vi "RIOTargetUI.vi"() -> ()   [LabVIEW 2014, in "RIO Target.lvclass"]
doc: "UI that will be called when the node is selected."
uses:
  RIO Target/RIO Target.lvclass
  <vilib>/NI/Configuration Framework/Node/NodeRef.ctl
  <vilib>/NI/Configuration Framework/Node/NISE_CEF_Node.lvclass
  <vilib>/NI/AMC/Message Queue.ctl
  <vilib>/NI/AMC/Message.ctl
  <vilib>/NI/Tools/Keyed Array/KeyedArray.ctl
  <vilib>/NI/Configuration Framework/Node/UserEventRef.ctl
  <vilib>/NI/Configuration Framework/Controls/EventCluster.ctl
  RIO Target/RIO Target.lvclass/RIO Target.ctl
  <vilib>/NI/Configuration Framework/serializable configuration/set metadata property.vi
  RIO Target Configuration/RIO Target Configuration.lvclass
  <vilib>/NI/Tools/Keyed Array/Tools_KeyedArray.lvlib
  <vilib>/NI/AMC/AMC.lvlib
  <vilib>/NI/Configuration Framework/NISE_CEF_TreeControl.lvlib
panel:
  out "error out":errorcluster
  in  "VI to Place Engines and IO Nodes":path
  in  "Destination Path":path
  in  "Target Project Path":path
  out "Channels per Device":string[][](table)
  in  "Generate":bool
  in  "user event":T1
  in  "main queue":T2
  in  "node ref":T3
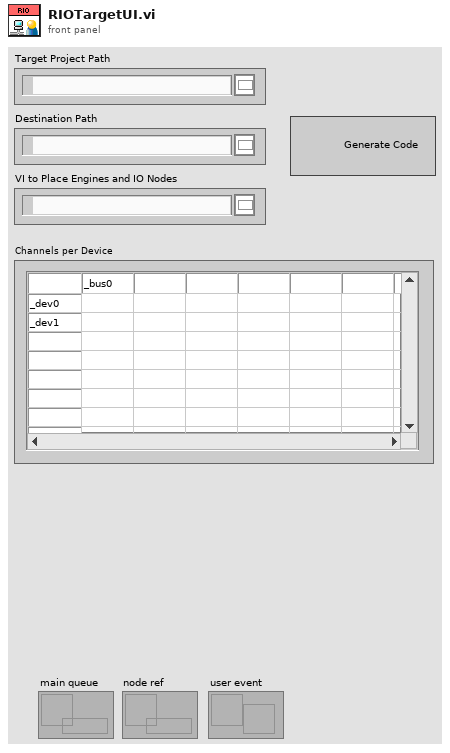
[diagram p1: front panel]
types:
  T1 = typedef "NISE_CEF_Node.lvclass/UserEventRef.ctl" = refnum<user-event>
  T2 = typedef "AMC.lvlib/Message Queue.ctl" = refnum<queue>
  T3 = typedef "NISE_CEF_Node.lvclass/NodeRef.ctl" = refnum<data-value>
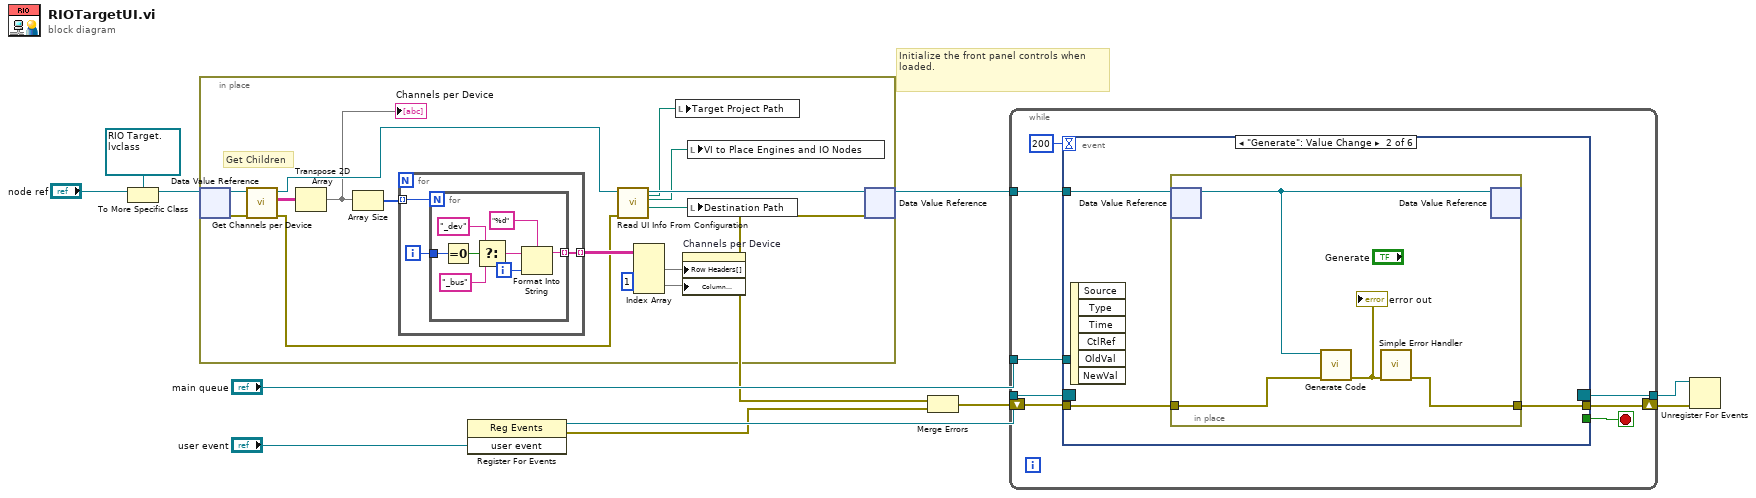
[diagram p0: block diagram]
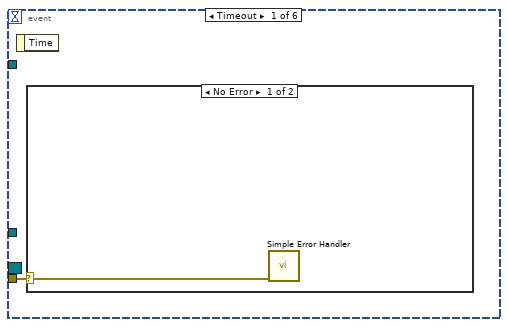
[diagram p2: hidden frame]
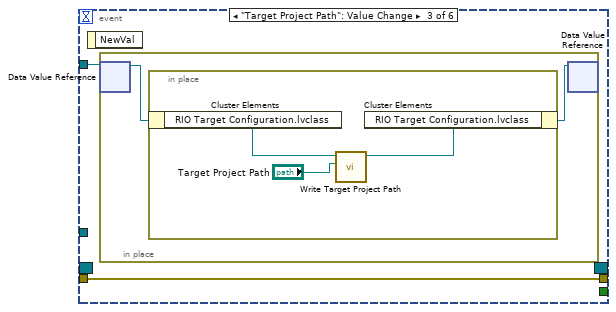
[diagram p4: hidden frame]
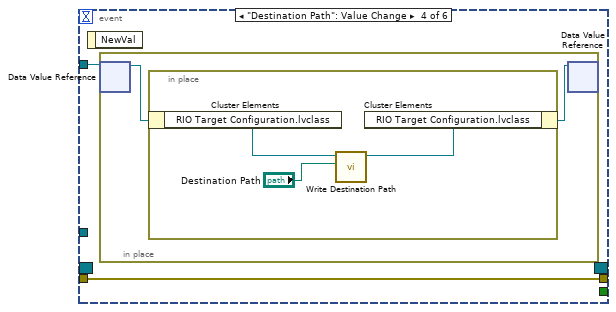
[diagram p5: hidden frame]
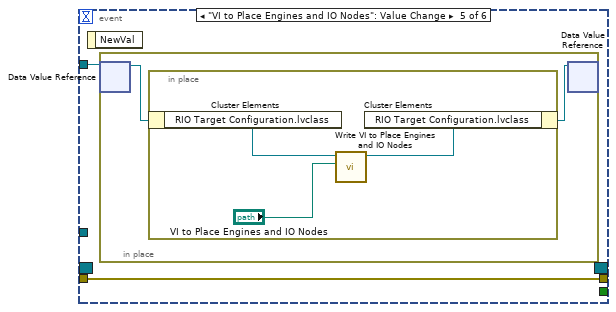
[diagram p6: hidden frame]
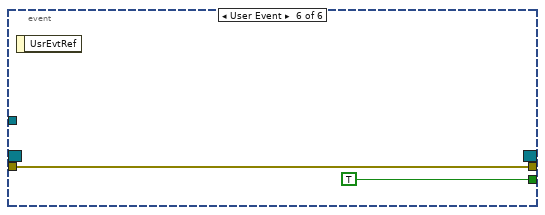
[diagram p7: hidden frame]
diagram:
  # "Initialize the front panel controls when loaded."
  n1 = To More Specific Class(target class=refnum<data-value> refnum ("data value reference"), reference="node ref") -> (specific class reference=w2:refnum<data-value>)  [unwired: 1 in, 1 out]
  n2 = in-place {
    # "Get Children"
    n3 = in-place-dvr #1(w2) -> (w18:refnum<class "RIO Target.lvclass">, w14:errorcluster)
    n4 = call "Get Channels per Device.vi"("error in (no error)"=w14, "RIO Target in"=w18) -> ("error out"=w13:errorcluster, "Channels per Device"=w17:string[][], "RIO Target out"=w16:refnum<class "RIO Target.lvclass">)  [unwired: 7 in]
    n5 = Transpose 2D Array(2D array=w17) -> (transposed array=w15:string[][])
    "Channels per Device" <- w15
    n6 = Array Size(array=w15) -> (size(s)=w27:i32[])
    n7 = for {
      tunnel: w27 -> [w30] mode=indexing
      tunnel: [w28] -> w26 mode=indexing
      i -> [w29]
      n8 = for {
        N: w30 -> [_]
        tunnel: w29 -> [w38]
        tunnel: [w31] -> w28 mode=indexing
        i -> [w32]
        n9 = Equal To 0?(x=w38) -> (x = 0?=w37:bool)
        n10 = Select(t="_dev", s=w37, f="_bus") -> (s? t:f=w34:string)
        n11 = Format Into String(format string="%d", initial string=w34, w32) -> (resulting string=w31:string)  [unwired: 1 in, 1 out]
      }
    }
    n12 = call "Read UI Info From Configuration.vi"("error in (no error)"=w13, "node in"=w16) -> ("Destination Path"=w19:path, "VI to Place Engines and IO Nodes"=w20:path, "node out"=w22:refnum<class "RIO Target.lvclass">, "Target Project Path"=w21:path)  [unwired: 5 in, 1 out]
    n13 = Index Array(array=w26, index (row) #2=1 ("index (row)")) -> (element #1=w24:string[], element #2=w23:string[])  [unwired: 3 in]
    n14 = local write "Target Project Path"(w21) -> ()
    n15 = property on="Channels per Device" class="Tbl (strict)"("Row Headers[]"=w24, "Column Headers[]"=w23) -> ()  [unwired: 2 in, 2 out]
    n16 = local write "VI to Place Engines and IO Nodes"(w20) -> ()
    n17 = local write "Destination Path"(w19) -> ()
    n18 = in-place-dvr #1(w22) -> (w12:refnum<data-value>, w6:errorcluster)
  }
  n19 = register-events("user event") -> (reference out=w9:refnum<event-registration>, error out=w1:errorcluster)  [unwired: 2 in]
  n20 = Merge Errors(w6, w1) -> (w5:errorcluster)
  n21 = while {
    tunnel: w12 -> [w46]
    tunnel: "main queue" -> [w45]
    tunnel: w9 -> [w43]
    tunnel: [w42] -> w8
    shift-right: [w40] -> w7
    shift-left: w5 -> [w39]
    stop <- w41 stop-if-true
    n22 = event shown="[1] \"Generate\": Value Change" {
      selector: w43 -> [_ _ _ _ _ _]
      dyn-events: [_ _ _ _ _ _] -> w42
      timeout: 200 -> [_ _ _ _ _ _]
      tunnel: w46 -> [_ w49 w56 w63 w70 _]
      tunnel: w45 -> [_ _ _ _ _ _]
      tunnel: [_ _ _ _ _ TRUE] -> w41
      tunnel: [_ w50 w57 w64 w71 w77] -> w40
      tunnel: w39 -> [w47 w51 w57 w64 w71 w77]
      event Timeout {
        n23 = event-data() -> ()  [unwired: 1 in, 1 out]
        n24 = case shown="No Error" w47 {
          selector: w47 -> [w48 _]
          frame No Error {
            n25 = call <vilib>:"Simple Error Handler.vi"("error in (no error)"=w48) -> ()  [unwired: 4 in, 5 out]
          }
          frame Error {
          }
        }
      }
      event "Generate": Value Change {
        n26 = event-data() -> ()  [unwired: 1 in, 6 out]
        n27 = in-place {
          in-place-border: w51 -> [w55]
          in-place-border: [w52] -> w50
          n28 = in-place-dvr #2(w49) -> (w54:refnum<class "RIO Target.lvclass">)  [unwired: 1 out]
          n29 = call "Generate Code.vi"("error in"=w55, "node in"=w54) -> ("error out"=w53:errorcluster)  [unwired: 9 in]
          "error out" <- w53
          n30 = call <vilib>:"Simple Error Handler.vi"("error in (no error)"=w53) -> ("error out"=w52:errorcluster)  [unwired: 4 in, 4 out]
          n31 = in-place-dvr #2(w54) -> ()  [unwired: 2 out]
        }
      }
      event "Target Project Path": Value Change {
        n32 = event-data() -> ()  [unwired: 1 in, 1 out]
        n33 = in-place {
          n34 = in-place-dvr #3(w56) -> (w59:refnum<class "RIO Target.lvclass">)  [unwired: 1 out]
          n35 = in-place {
            n36 = in-place-cluster #4(w59) -> ("RIO Target Configuration.lvclass"=w62:refnum<class "RIO Target Configuration.lvclass">)
            n37 = call "Write Target Project Path.vi"("Target Project Path"="Target Project Path", "RIO Target Configuration in"=w62) -> ("RIO Target Configuration out"=w61:refnum<class "RIO Target Configuration.lvclass">)  [unwired: 8 in, 1 out]
            n38 = in-place-cluster #4("RIO Target Configuration.lvclass"=w61) -> (w58:refnum<class "RIO Target.lvclass">)
          }
          n39 = in-place-dvr #3(w58) -> ()  [unwired: 2 out]
        }
      }
      event "Destination Path": Value Change {
        n40 = event-data() -> ()  [unwired: 1 in, 1 out]
        n41 = in-place {
          n42 = in-place-dvr #5(w63) -> (w66:refnum<class "RIO Target.lvclass">)  [unwired: 1 out]
          n43 = in-place {
            n44 = in-place-cluster #6(w66) -> ("RIO Target Configuration.lvclass"=w69:refnum<class "RIO Target Configuration.lvclass">)
            n45 = call "Write Destination Path.vi"("Destination Path"="Destination Path", "RIO Target Configuration in"=w69) -> ("RIO Target Configuration out"=w68:refnum<class "RIO Target Configuration.lvclass">)  [unwired: 8 in, 1 out]
            n46 = in-place-cluster #6("RIO Target Configuration.lvclass"=w68) -> (w65:refnum<class "RIO Target.lvclass">)
          }
          n47 = in-place-dvr #5(w65) -> ()  [unwired: 2 out]
        }
      }
      event "VI to Place Engines and IO Nodes": Value Change {
        n48 = event-data() -> ()  [unwired: 1 in, 1 out]
        n49 = in-place {
          n50 = in-place-dvr #7(w70) -> (w73:refnum<class "RIO Target.lvclass">)  [unwired: 1 out]
          n51 = in-place {
            n52 = in-place-cluster #8(w73) -> ("RIO Target Configuration.lvclass"=w76:refnum<class "RIO Target Configuration.lvclass">)
            n53 = call "Write VI to Place Engines and IO Nodes.vi"("VI to Place Engines and IO Nodes"="VI to Place Engines and IO Nodes", "RIO Target Configuration in"=w76) -> ("RIO Target Configuration out"=w75:refnum<class "RIO Target Configuration.lvclass">)  [unwired: 8 in, 1 out]
            n54 = in-place-cluster #8("RIO Target Configuration.lvclass"=w75) -> (w72:refnum<class "RIO Target.lvclass">)
          }
          n55 = in-place-dvr #7(w72) -> ()  [unwired: 2 out]
        }
      }
      event User Event {
        n56 = event-data() -> ()  [unwired: 1 in, 1 out]
      }
    }
  }
  n57 = Unregister For Events(event registration refnum=w8, error in=w7) -> ()  [unwired: 1 out]
